vi "DB - [AMS].[Execute].[EventLog].vi"(5 "DB - [AMS].[Execute].[EventLog]":T1=enum."INSERT", 7 "DB Connection":T4={"Open"=TRUE, "Close"=TRUE}, 8 "error in (no error)":errorcluster, 10 "AMS Execute EventLog":T2, 11 "connection reference":T3) -> (0 "SUMMARY":errorcluster, 1 "time stamp":timestamp format="%<%I:%M:%S%3u %p\n%x>T", 2 "[CreatedOn]":string, 3 "connection reference":T3, 4 "[LastMessageNo]":string)   [LabVIEW 2013]
doc: "Array (0xFFFE autodetect)\n ([EventType]\n ,[Source]\n ,[UserId]\n ,[Computer]\n ,[CreatedOn])"
uses:
  <vilib>/addons/database/Connection.llb/Conn ObjectReference.ctl
  Controls/DB - OpenClose.ctl
  Controls/DB - AMS Execute EventLog.ctl
  Controls/DB - [AMS].[Execute].[EventLog] Enum.ctl
  Controls/Global AMS.vi
  Controls/Global SRTRS.vi
  <vilib>/addons/database/Connection.llb/DB Tools Open Connec (String).vi
  <vilib>/addons/database/Connection.llb/Conn Execute.vi
  <vilib>/addons/database/Recordset.llb/Rec Destroy - Connection.vi
  <vilib>/addons/database/NI_Database_API.lvlib
panel:
  out "Close":errorcluster
  out "SQL Statement":string
  in  "AMS.Execute.EventLog":string="AMS.Execute.EventLog"
  out "Connection Information":T5={"Connection "="SQL Server 32bit HPEnvy", "Username"="admin", "Password"="admin123"}
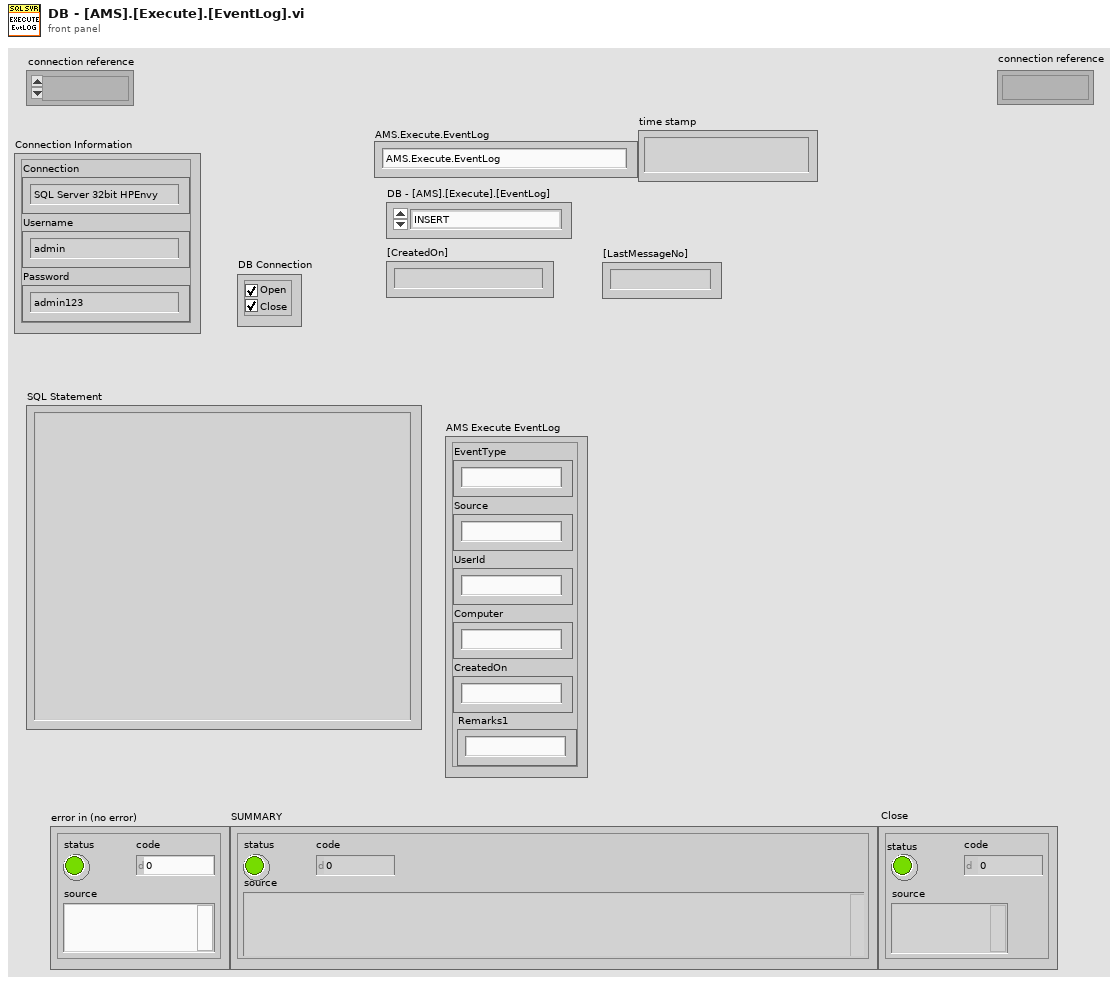
[diagram p1: front panel]
types:
  T1 = typedef "DB - [AMS].[Execute].[EventLog] Enum.ctl" = enum16{"SELECT 'CreatedOn'", "SELECT 'LastMessageNo'", "INSERT"}
  T2 = typedef "DB - AMS Execute EventLog.ctl" = cluster{"EventType":string, "Source":string, "UserId":string, "Computer":string, "CreatedOn":string, "Remarks1":string}
  T3 = typedef "NI_Database_API.lvlib/Conn ObjectReference.ctl" = refnum<k1>
  T4 = typedef "DB - OpenClose.ctl" = cluster{"Open":bool, "Close":bool}
  T5 = cluster{"Connection ":string, "Username":string, "Password":string}
  T6 = typedef "Enum - InteractiveMode-SubVIMode.ctl" = enum16{"Interactive", "subVI Mode"}
  T7 = typedef "Connection Information Cluster.ctl" = cluster{"Connection ":string, "Username":string, "Password":string}
  T8 = typedef "DB - DB.Schema.Table.ctl" = cluster{"DB":string, "Schema":string, "Table":string}
  T9 = typedef "NI_Database_API.lvlib/Rec ObjectReference.ctl" = refnum<k1>
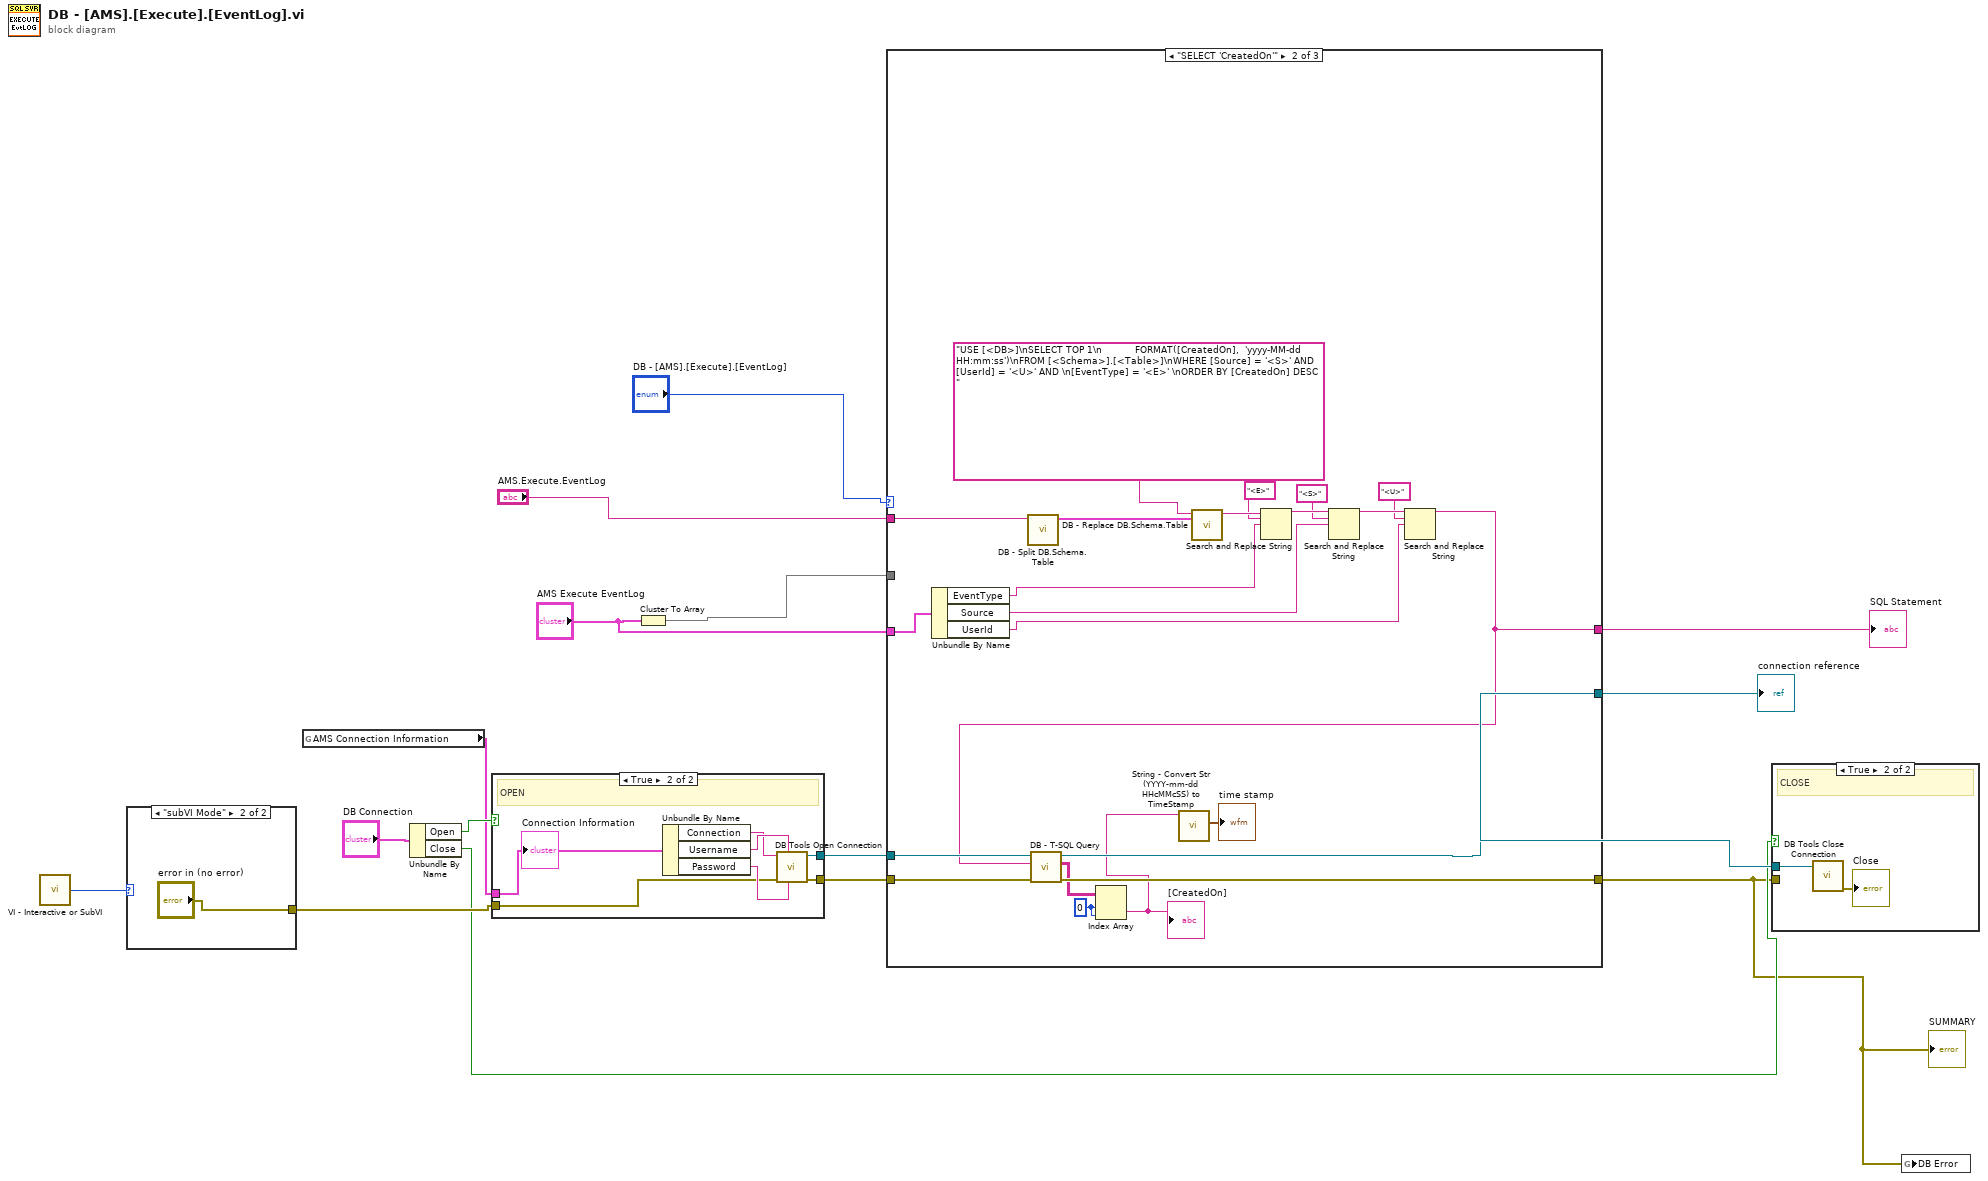
[diagram p0: block diagram]
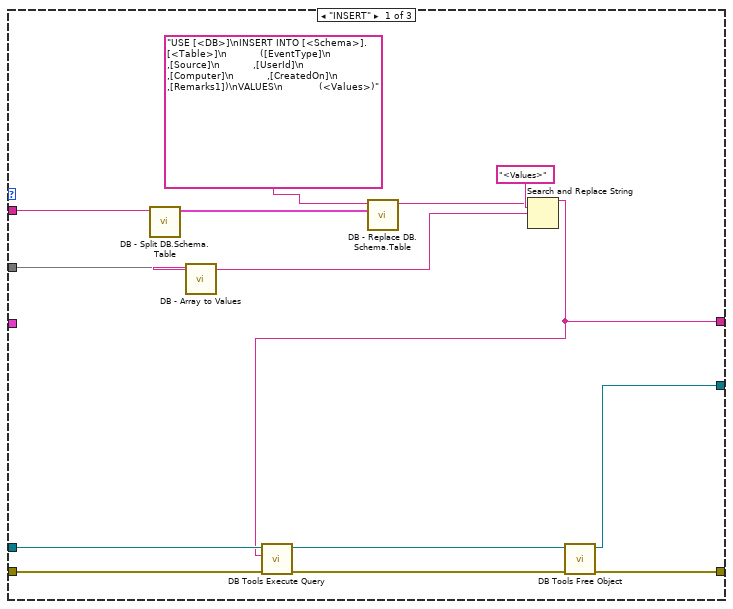
[diagram p2: hidden frame]
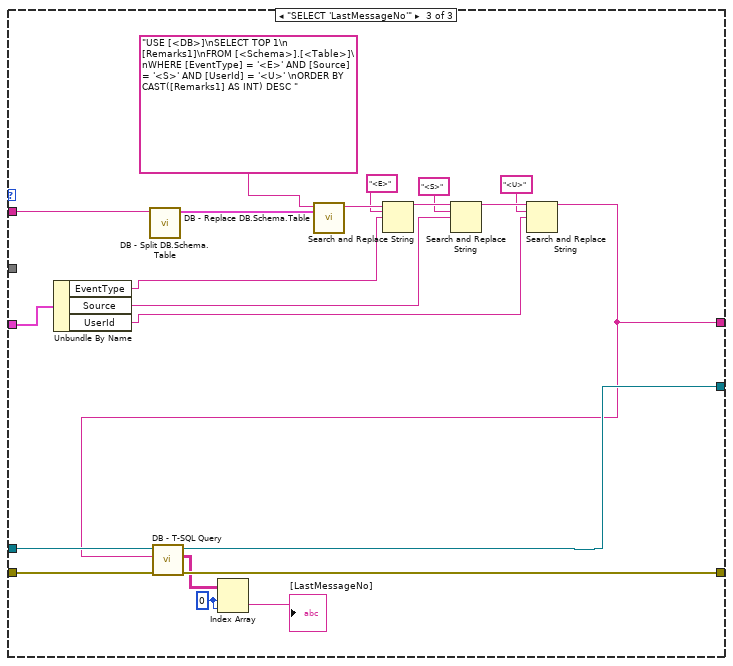
[diagram p3: hidden frame]
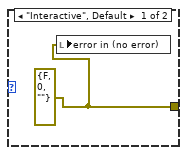
[diagram p5: hidden frame]
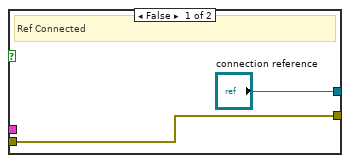
[diagram p6: hidden frame]
diagram:
  n1 = call "VI - Interactive or SubVI.vi"() -> ("Mode"=w13:T6)  [unwired: 5 in]
  n2 = case shown="\"subVI Mode\"" w13 {
    tunnel: [w16 "error in (no error)"] -> w12
    frame "Interactive", Default {
      w16 = errorcluster {"status"=FALSE, "code"=0, "source"=""} ("error in (no error)")
      n3 = local write "error in (no error)"(w16) -> ()
    }
    frame "subVI Mode" {
    }
  }
  n4 = global read "Global AMS.vi" "AMS Connection Information"() -> (w5:T7)
  n5 = Unbundle By Name("DB Connection") -> ("Open"=w14:bool, "Close"=w8:bool)
  n6 = case shown="True" w14 {
    tunnel: ["connection reference" w23] -> w11
    tunnel: w12 -> [w18 w22]
    tunnel: [w18 w21] -> w10
    tunnel: w5 -> [_ w20]
    frame False {
      # "Ref Connected"
    }
    frame True {
      # "OPEN"
      n7 = Unbundle By Name(w20) -> ("Connection"=w25:string, "Username"=w26:string, "Password"=w24:string)
      n8 = call-poly <vilib>:"DB Tools Open Connection.vi"("password"=w24, "userID"=w26, "error in (no error)"=w22, "connection information"=w25) -> ("error out"=w21:errorcluster, "connection reference"=w23:T3)  [unwired: 4 in]
      "Connection Information" <- w20
    }
  }
  n9 = Cluster To Array(cluster="AMS Execute EventLog") -> (array=w3:string[])
  n10 = case shown="\"SELECT 'CreatedOn'\"" "DB - [AMS].[Execute].[EventLog]" {
    tunnel: w11 -> [w40 w59 w80]
    tunnel: w10 -> [w39 w58 w79]
    tunnel: [w38 w56 w77] -> w9
    tunnel: [w36 w57 w78] -> w7
    tunnel: "AMS.Execute.EventLog" -> [w35 w61 w82]
    tunnel: [w30 w48 w69] -> w4
    tunnel: w3 -> [w27 _ _]
    tunnel: "AMS Execute EventLog" -> [_ w51 w72]
    frame "INSERT" {
      n11 = call "DB - Split DB.Schema.Table.vi"("DB.Schema.Table"=w35) -> ("DB.Schema.Table"=w37:T8)  [unwired: 10 in]
      n12 = call "DB - Array to Values.vi"("Array (0xFFFE autodetect)"=w27) -> ("<Values>"=w31:string)  [unwired: 10 in]
      n13 = call "DB - Replace DB.Schema.Table.vi"("DB.Schema.Table"=w37, "string in"="USE [<DB>]\nINSERT INTO [<Schema>].[<Table>]\n           ([EventType]\n           ,[Source]\n           ,[UserId]\n           ,[Computer]\n           ,[CreatedOn]\n           ,[Remarks1])\nVALUES\n            (<Values>)") -> ("string out"=w32:string)  [unwired: 8 in, 1 out]
      n14 = Search and Replace String(input string=w32, search string="<Values>", replace string=w31) -> (result string=w30:string)  [unwired: 5 in, 3 out]
      n15 = call-poly <vilib>:"DB Tools Execute Query.vi"("error in (no error)"=w39, "SQL query"=w30, "connection reference"=w40) -> ("error out"=w28:errorcluster, "recordset reference"=w29:T9)  [unwired: 5 in]
      n16 = call-poly <vilib>:"DB Tools Free Object.vi"("error in (no error)"=w28, "recordset reference"=w29) -> ("error out"=w36:errorcluster, "connection reference"=w38:T3)  [unwired: 8 in]
    }
    frame "SELECT 'CreatedOn'" {
      w54 = 0 ("index (row)")
      n17 = Unbundle By Name(w51) -> ("EventType"=w47:string, "Source"=w46:string, "UserId"=w43:string)
      n18 = call "DB - Split DB.Schema.Table.vi"("DB.Schema.Table"=w61) -> ("DB.Schema.Table"=w62:T8)  [unwired: 10 in]
      n19 = call "DB - Replace DB.Schema.Table.vi"("DB.Schema.Table"=w62, "string in"="USE [<DB>]\nSELECT TOP 1\n           FORMAT([CreatedOn],  'yyyy-MM-dd HH:mm:ss')\nFROM [<Schema>].[<Table>]\nWHERE [Source] = '<S>' AND [UserId] = '<U>' AND \n[EventType] = '<E>' \nORDER BY [CreatedOn] DESC ") -> ("string out"=w53:string)  [unwired: 8 in, 1 out]
      n20 = Search and Replace String(input string=w53, search string="<E>", replace string=w47) -> (result string=w50:string)  [unwired: 5 in, 3 out]
      n21 = Search and Replace String(input string=w50, search string="<S>", replace string=w46) -> (result string=w49:string)  [unwired: 5 in, 3 out]
      n22 = Search and Replace String(input string=w49, search string="<U>", replace string=w43) -> (result string=w48:string)  [unwired: 5 in, 3 out]
      n23 = call "DB - T-SQL Query.vi"("error in (no error)"=w58, "T-SQL"=w48, "connection reference"=w59) -> ("error out"=w57:errorcluster, "2D data"=w55:string[][], "connection reference"=w56:T3)  [unwired: 6 in]
      n24 = Index Array(array=w55, index (row)=w54, index (col)=w54) -> (element=w42:string)
      "[CreatedOn]" <- w42
      n25 = call "String - Convert Str (YYYY-mm-dd HHcMMcSS) to TimeStamp.vi"("YYYY-mm-dd HH:MM:SS (String)"=w42) -> ("time stamp"=→"time stamp":timestamp)  [unwired: 9 in, 1 out]
    }
    frame "SELECT 'LastMessageNo'" {
      w75 = 0 ("index (row)")
      n26 = Unbundle By Name(w72) -> ("EventType"=w68:string, "Source"=w67:string, "UserId"=w64:string)
      n27 = call "DB - Split DB.Schema.Table.vi"("DB.Schema.Table"=w82) -> ("DB.Schema.Table"=w83:T8)  [unwired: 10 in]
      n28 = call "DB - Replace DB.Schema.Table.vi"("DB.Schema.Table"=w83, "string in"="USE [<DB>]\nSELECT TOP 1\n          [Remarks1]\nFROM [<Schema>].[<Table>]\nWHERE [EventType] = '<E>' AND [Source] = '<S>' AND [UserId] = '<U>' \nORDER BY CAST([Remarks1] AS INT) DESC ") -> ("string out"=w74:string)  [unwired: 8 in, 1 out]
      n29 = Search and Replace String(input string=w74, search string="<E>", replace string=w68) -> (result string=w71:string)  [unwired: 5 in, 3 out]
      n30 = Search and Replace String(input string=w71, search string="<S>", replace string=w67) -> (result string=w70:string)  [unwired: 5 in, 3 out]
      n31 = Search and Replace String(input string=w70, search string="<U>", replace string=w64) -> (result string=w69:string)  [unwired: 5 in, 3 out]
      n32 = call "DB - T-SQL Query.vi"("error in (no error)"=w79, "T-SQL"=w69, "connection reference"=w80) -> ("error out"=w78:errorcluster, "2D data"=w76:string[][], "connection reference"=w77:T3)  [unwired: 6 in]
      n33 = Index Array(array=w76, index (row)=w75, index (col)=w75) -> (element=→"[LastMessageNo]":string)
    }
  }
  "SUMMARY" <- w7
  "connection reference" <- w9
  "SQL Statement" <- w4
  n34 = case shown="True" w8 {
    tunnel: w9 -> [_ w85]
    tunnel: w7 -> [_ _]
    frame False {
      # "Ref Connected"
    }
    frame True {
      # "CLOSE"
      n35 = call <vilib>:"DB Tools Close Connection.vi"("connection reference"=w85) -> ("error out"=→"Close":errorcluster)  [unwired: 6 in]
    }
  }
  n36 = global write "Global SRTRS.vi" "DB Error"(w7) -> ()
